vi "Image Process.vi"() -> (0 "Motor Output":dbl=0.96, 2 "Image Out 3":T1(plugin-control), 3 "Bandwidth (kbps)":dbl=4.83399006772009)   [LabVIEW 2012]
uses:
  <vilib>/Rock Robotics/WPI/Camera/WPI_CameraImageSize.ctl
  <vilib>/addons/control/pid/pid.llb/PID (DBL).vi
  <vilib>/addons/control/pid/NI_PID_pid.lvlib
panel:
  out "Particle Measurements (Pixels)":dbl[][](array[numeric]) format="%.2f"
  out "error out":errorcluster
  out "String":string="0.960000"
  in  "Vision PID limits":cluster{"output high":dbl, "output low":dbl}={"output high"=1.0, "output low"=-1.0} {"output low" format="%.2f"; "output high" format="%.2f"}
  in  "Vision PID gains":T2={"proportional gain (Kc)"=0.003, "integral time (Ti, min)"=0.0, "derivative time (Td, min)"=0.0} {"derivative time (Td, min)" format="%.3f"; "integral time (Ti, min)" format="%.3f"; "proportional gain (Kc)" format="%.3f"}
  # "P= 0.003\nI = 0\nD = 0"
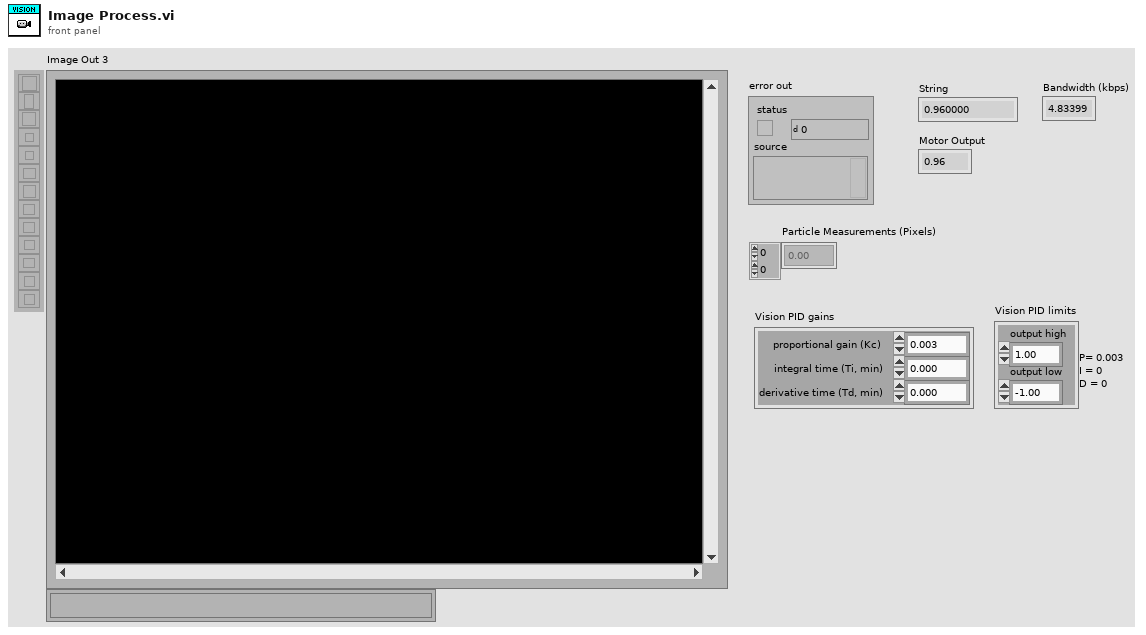
[diagram p1: front panel]
types:
  T1 = typedef "IMAQ Image.ctl" = refnum<image>
  T2 = cluster{"proportional gain (Kc)":dbl, "integral time (Ti, min)":dbl, "derivative time (Td, min)":dbl}
  T3 = typedef "Image Type" = u32
  T4 = typedef "WPI_CameraImageSize.ctl" = enum16{"640x480", "320x240", "160x120"}
  T5 = cluster{"fps":i32, "compression":i32, "Image Size":T4}
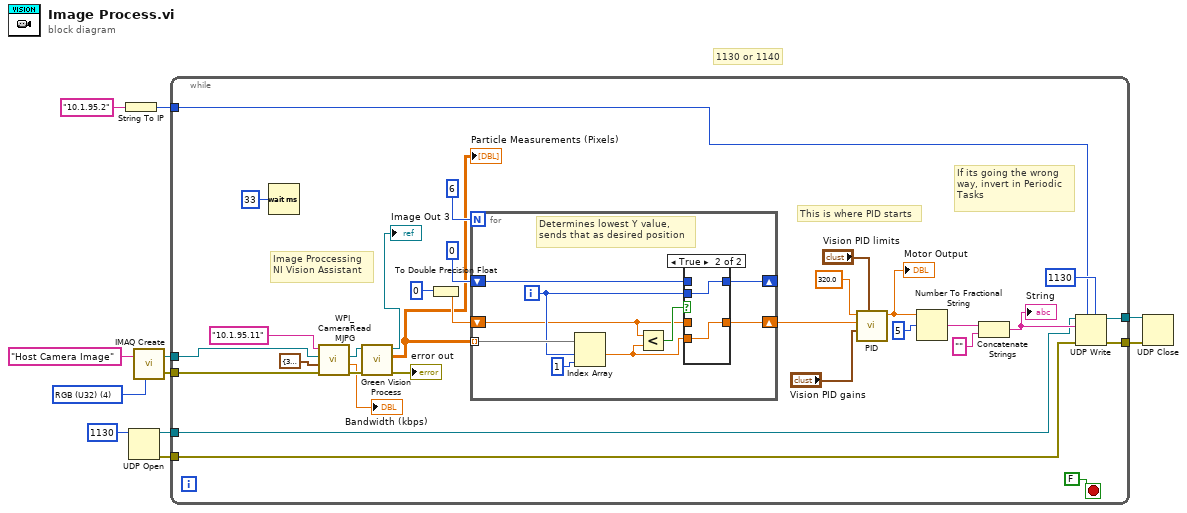
[diagram p0: block diagram]
diagram:
  w4 = T3 4 items=["Grayscale (U8)", "Grayscale (I16)", "Grayscale (SGL)", "Complex (CSG)", "RGB (U32)", "HSL (U32)", "RGB (U64)"] ("Image Type")
  # "1130 or 1140"
  n1 = String To IP(1:"10.1.95.2" ("name")) -> (0:w5:u32)
  n2 = UDP Open(11:u16 1130 ("port")) -> (port=w10:refnum<k16>, 0:w9:errorcluster)  [unwired: 4 in, 1 out]
  n3 = call "IMAQ Create"("Image Name"="Host Camera Image", "Image Type"=w4) -> ("New Image"=w1:T1, "error out"=w2:errorcluster)  [unwired: 2 in, 1 out]
  n4 = while {
    tunnel: w10 -> [w12]
    tunnel: w9 -> [w19]
    tunnel: [w32] -> w8
    tunnel: [w33] -> w7
    tunnel: w5 -> [w30]
    tunnel: w2 -> [w22]
    tunnel: w1 -> [w21]
    stop <- FALSE stop-if-true
    # "If its going the wrong\nway, invert in Periodic\nTasks"
    # "Image Proccessing\nNI Vision Assistant"
    # "This is where PID starts"
    n5 = Wait (ms)(milliseconds to wait=u32 33) -> ()  [unwired: 1 out]
    n6 = call <vilib>:"WPI_CameraRead MJPG.vi"("error in"=w22, "Camera Settings"=T5 {"fps"=30, "compression"=30, "Image Size"=enum."640x480"}, "Image"=w21, "address"="10.1.95.11" ("Robot IP Address")) -> ("error out"=w24:errorcluster, "Bandwidth (kbps)"=→"Bandwidth (kbps)":dbl, "Image Out"=w25:T1)  [unwired: 5 in]
    n7 = call "Green Vision Process.vi"("error in (no error)"=w24, "Refnum in"=w25) -> ("error out"=→"error out":errorcluster, "Particle Measurements (Pixels)"=w20:dbl[][], "Refnum out"=→"Image Out 3":T1)  [unwired: 6 in, 1 out]
    "Particle Measurements (Pixels)" <- w20
    n8 = To Double Precision Float(number=0) -> (double precision float=w36:dbl)
    n9 = for {
      N: 6 -> [_]
      tunnel: w20 -> [w50] mode=indexing
      shift-right: [w47] -> w35
      shift-left: w36 -> [w43]
      shift-right: [w46] -> _
      shift-left: 0 -> [w48]
      i -> [w49]
      # "Determines lowest Y value,\nsends that as desired position"
      n10 = Index Array(array=w50, index #1=w49, index #2=1 ("disabled index (col)")) -> (element #1=w44:dbl)  [unwired: 1 out]
      n11 = Less?(x=w43, y=w44) -> (x < y?=w51:bool)
      n12 = case shown="True" w51 {
        tunnel: w49 -> [_ w55]
        tunnel: [w52 w55] -> w46
        tunnel: w44 -> [_ w54]
        tunnel: [w53 w54] -> w47
        tunnel: w43 -> [w53 _]
        tunnel: w48 -> [w52 _]
        frame False {
        }
        frame True {
        }
      }
    }
    n13 = call-poly <vilib>:"PID.vi"("output range"="Vision PID limits", "PID gains"="Vision PID gains", "process variable"=w35, "setpoint"=320.0) -> ("output"=w16:dbl)  [unwired: 6 in, 1 out]
    "Motor Output" <- w16
    n14 = Number To Fractional String(number=w16, width (-)=i16 5) -> (F-format string=w14:string)  [unwired: 2 in]
    n15 = Concatenate Strings(w14, "" ("string")) -> (w28:string)
    "String" <- w28
    n16 = UDP Write(address=w30, port or service name=u16 1130, connection ID=w12, data in=w28, 8:w19) -> (error out=w32:errorcluster, 3:w33:refnum<k16>)  [unwired: 1 in]
  }
  n17 = UDP Close(connection ID=w7, 8:w8) -> ()  [unwired: 2 out]
